vi "Read First Character.vi"(8 "Error In":errorcluster) -> (0 "Error Out":errorcluster)   [LabVIEW 2018, in "Tests.lvlib" / "Readers.lvlib" / "String.lvlib"]
uses:
  String.lvlib
  src/Toolkit/Readers/String/String.lvclass
  <vilib>/addons/_JKI Toolkits/Caraya/classes/Test/Test.lvclass
  <vilib>/addons/_JKI Toolkits/Caraya/classes/Assert/Assert.lvclass
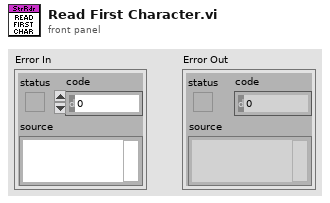
[diagram p1: front panel]
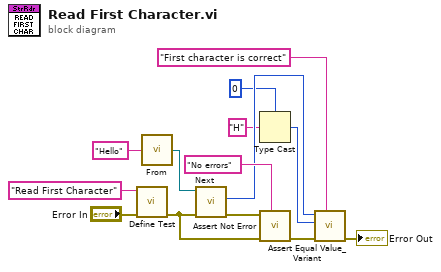
[diagram p0: block diagram]
diagram:
  n1 = call <vilib>:"Define Test.vi"("error in (no error)"="Error In", "Label (VI Title)"="Read First Character") -> ("error out"=w1:errorcluster)  [unwired: 9 in]
  n2 = call "From.vi"("String"="Hello") -> ("String"=w11:refnum<class "String.lvclass">)
  n3 = call-dynamic "Next.vi"("Error In"=w1, "Reader In"=w11) -> ("Error Out"=w10:errorcluster, "Character"=w6:u8)  [unwired: 6 in, 2 out]
  n4 = Type Cast(type=u8 0, x="H") -> (*(type *) &x=w2:u8)
  n5 = call <vilib>:"Assert Not Error.vi"("Label"="No errors", "error in (no error)"=w1, "Not Error?"=w10) -> ("error out"=w8:errorcluster)  [unwired: 8 in]
  n6 = call <vilib>:"Assert Equal Value_Variant.vi"("Label"="First character is correct", "error in (no error)"=w8, "Y"=w2, "X"=w6) -> ("error out"=→"Error Out":errorcluster)  [unwired: 7 in]
